vi "AddNoise.vi"(10 "Noise Level":dbl=0.01, 11 "In":dbl) -> (3 "Out":dbl)   [LabVIEW 2017]
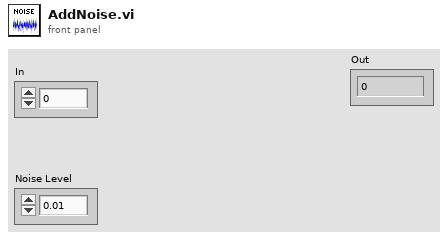
[diagram p1: front panel]
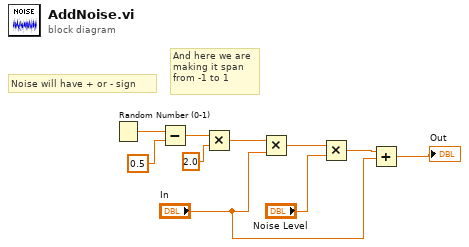
[diagram p0: block diagram]
diagram:
  # "And here we are\nmaking it span \nfrom -1 to 1"
  # "Noise will have + or - sign"
  n1 = Random Number (0-1)() -> (number: 0 to 1=w10:dbl)
  n2 = Subtract(x=w10, y=0.5) -> (x-y=w6:dbl)
  n3 = Multiply(x=w6, y=2.0) -> (x*y=w4:dbl)
  n4 = Multiply(x=w4, y="In") -> (x*y=w8:dbl)
  n5 = Multiply(x=w8, y="Noise Level") -> (x*y=w3:dbl)
  n6 = Add(x=w3, y="In") -> (x+y=→"Out":dbl)
